vi "Print AutoCal FP.vi"(10 "name or relative path":string, 11 "VI in":refnum<vi>) -> ()   [LabVIEW 2015]
uses:
  <vilib>/printing/EasyPrintingControls.llb/layout_options.ctl
  <vilib>/printing/EasyPrintingControls.llb/orientation.ctl
  <vilib>/printing/EasyPrintingControls.llb/panel_scaling_for_page.ctl
  <vilib>/printing/EasyPrintingControls.llb/margins.ctl
  <vilib>/printing/EasyPrintingControls.llb/margin_values.ctl
  <vilib>/printing/EasyPrintingControls.llb/measurement_system.ctl
  <vilib>/printing/EasyPrintingControls.llb/printer_options.ctl
  <vilib>/printing/EasyPrintingControls.llb/printing_method.ctl
  <vilib>/printing/EasyPrintingControls.llb/color_or_monochrome.ctl
  <vilib>/printing/EasyPrintingControls.llb/page_header_options.ctl
  <vilib>/printing/EasyPrintingControls.llb/page_headers.ctl
  <vilib>/printing/EasyPrintingControls.llb/page_header_content_options.ctl
  <vilib>/printing/EasyPrinting.llb/Easy Print VI Panel or Documentation (refnum).vi
  <vilib>/Utility/NIReport.llb/NI_report.lvclass
  <vilib>/Utility/NIReport.llb/Append Image to Report (path wrap).vi
  <vilib>/Utility/NIReport.llb/NI_ReportGenerationCore.lvlib
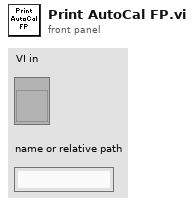
[diagram p1: front panel]
types:
  T1 = enum16{"Standard Report", "HTML", "Word", "Excel"}
  T2 = typedef "NI_ReportGenerationCore.lvlib/layout_options.ctl" = cluster{"orientation (unchanged)":T3, "panel scaling for page (unchanged)":T4, "margins":T5, "printer options":T8, "page header options":T11}
  T3 = typedef "NI_ReportGenerationCore.lvlib/orientation.ctl" = u16
  T4 = typedef "NI_ReportGenerationCore.lvlib/panel_scaling_for_page.ctl" = u16
  T5 = typedef "NI_ReportGenerationCore.lvlib/margins.ctl" = cluster{"override VI margins (false)":bool, "margins (1.00)":T6, "measurement system (default)":T7}
  T6 = typedef "NI_ReportGenerationCore.lvlib/margin_values.ctl" = cluster{"top":dbl, "left":dbl, "right":dbl, "bottom":dbl}
  T7 = typedef "NI_ReportGenerationCore.lvlib/measurement_system.ctl" = u16
  T8 = typedef "NI_ReportGenerationCore.lvlib/printer_options.ctl" = cluster{"destination printer name (current)":string, "printing method (unchanged)":T9, "color or monochrome (unchanged)":T10}
  T9 = typedef "NI_ReportGenerationCore.lvlib/printing_method.ctl" = u16
  T10 = typedef "NI_ReportGenerationCore.lvlib/color_or_monochrome.ctl" = u16
  T11 = typedef "NI_ReportGenerationCore.lvlib/page_header_options.ctl" = cluster{"page headers (unchanged)":T12, "page header content options":T13}
  T12 = typedef "NI_ReportGenerationCore.lvlib/page_headers.ctl" = u16
  T13 = typedef "NI_ReportGenerationCore.lvlib/page_header_content_options.ctl" = cluster{"Include VI Name":bool, "Include VI Path":bool, "Include Last Modification Date":bool, "Include Date Printed":bool, "Include Page Number":bool, "Include VI Icon":bool}
  T14 = typedef "imagedata.ctl" = cluster{"image type":i32, "image depth":i32, "image":u8[], "mask":u8[], "colors":u32[], "Rectangle":cluster{"left":i16, "top":i16, "right":i16, "bottom":i16}}
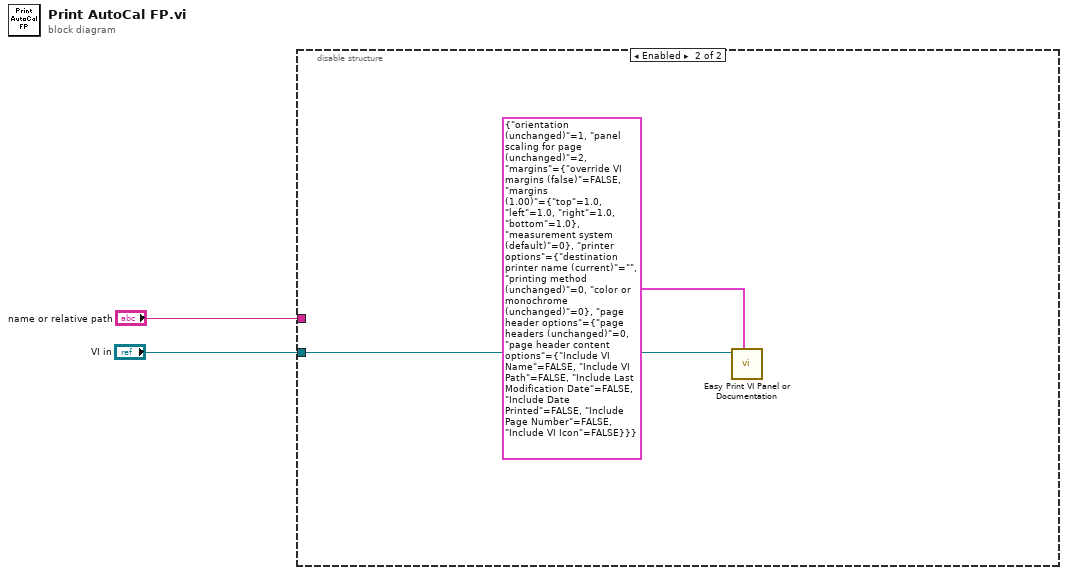
[diagram p0: block diagram]
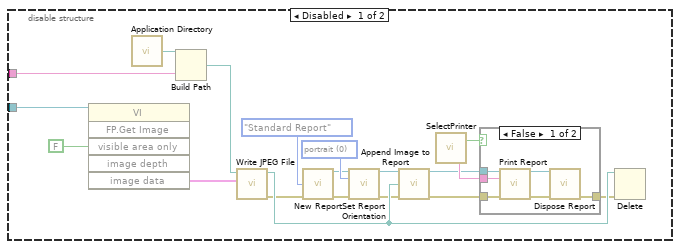
[diagram p2: hidden frame]
diagram:
  n1 = disable-structure shown="Enabled" {
    disable-tunnel: "name or relative path" -> [w7 _]
    disable-tunnel: "VI in" -> [w5 w30]
    frame Disabled {
      w16 = 0 items=["portrait", "landscape"] ("orientation (portrait)")
      n2 = invoke class="VI" method="FP.Get Image"(reference=w5, "visible area only"=FALSE ("Visible Area Only")) -> ("image data"=w4:T14)  [unwired: 4 in, 5 out]
      n3 = call <vilib>:"Application Directory.vi"() -> ("Application Directory"=w6:path)
      n4 = Build Path(base path=w6, name or relative path=w7) -> (appended path=w8:path)
      n5 = call <vilib>:"Write JPEG File.vi"("image data"=w4, "path to JPEG file"=w8) -> ("error out"=w19:errorcluster, "path"=w21:path)  [unwired: 1 in, 7 out]
      n6 = call <vilib>:"New Report.vi"("report type"=T1."Standard Report", "error in (no error)"=w19) -> ("report out"=w15:refnum<class "NI_report.lvclass">, "error out"=w11:errorcluster)  [unwired: 12 in]
      n7 = call-dynamic "Set Report Orientation.vi"("report in"=w15, "orientation (portrait)"=w16, "error in (no error)"=w11) -> ("report out"=w13:refnum<class "NI_report.lvclass">, "error out"=w10:errorcluster)  [unwired: 11 in]
      n8 = call-poly <vilib>:"Append Image to Report.vi"("report in"=w13, "path or URL of image"=w21, "error in (no error)"=w10) -> ("report out"=w12:refnum<class "NI_report.lvclass">, "error out"=w9:errorcluster)  [unwired: 9 in, 2 out]
      n9 = call "SelectPrinter.vi"() -> ("ChosenPrinter"=w17:string, "Closed?"=w18:bool)  [unwired: 2 in]
      n10 = case shown="False" w18 {
        tunnel: w12 -> [w27 _]
        tunnel: w17 -> [w25 _]
        tunnel: w9 -> [w24 w28]
        tunnel: [w22 w28] -> w20
        frame False {
          n11 = call-dynamic "Print Report.vi"("report in"=w27, "printer name (default)"=w25, "error in (no error)"=w24) -> ("report out"=w26:refnum<class "NI_report.lvclass">, "error out"=w23:errorcluster)  [unwired: 11 in]
          n12 = call-dynamic "Dispose Report.vi"("report in"=w26, "error in (no error)"=w23) -> ("error out"=w22:errorcluster)  [unwired: 13 in]
        }
        frame True {
        }
      }
      n13 = Delete(path (use dialog)=w21, error in=w20) -> ()  [unwired: 3 in, 3 out]
    }
    frame Enabled {
      n14 = call-poly <vilib>:"Easy Print VI Panel or Documentation.vi"("layout options"=T2 {"orientation (unchanged)"=1, "panel scaling for page (unchanged)"=2, "margins"={"override VI margins (false)"=FALSE, "margins (1.00)"={"top"=1.0, "left"=1.0, "right"=1.0, "bottom"=1.0}, "measurement system (default)"=0}, "printer options"={"destination printer name (current)"="", "printing method (unchanged)"=0, "color or monochrome (unchanged)"=0}, "page header options"={"page headers (unchanged)"=0, "page header content options"={"Include VI Name"=FALSE, "Include VI Path"=FALSE, "Include Last Modification Date"=FALSE, "Include Date Printed"=FALSE, "Include Page Number"=FALSE, "Include VI Icon"=FALSE}}}, "VI reference"=w30) -> ()  [unwired: 8 in, 2 out]
    }
  }
